vi "ConfigCalculateMinimalAcquisitionTime.vi"(7 "Single Pump Cycle Refresh Ratio":dbl, 9 "Loop Microscope Settings":string[][](array[string]), 10 "Positions":string[][](array[string]), 11 "Program":string[][](array[string])) -> (0 "Microscope Out":string[][](array[string]), 1 "Positions out":string[][](array[string]), 2 "Program out":string[][](array[string]), 3 "Time (Time Stamp)":timestamp)   [LabVIEW 2018, in "Config.lvlib"]
uses:
  Config.lvlib
  ContinuousLoop/ContinousLoop.lvlib
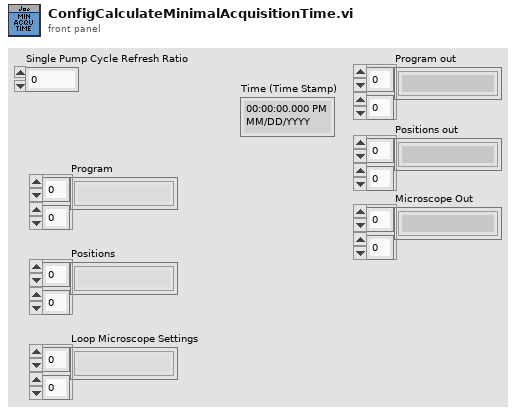
[diagram p1: front panel]
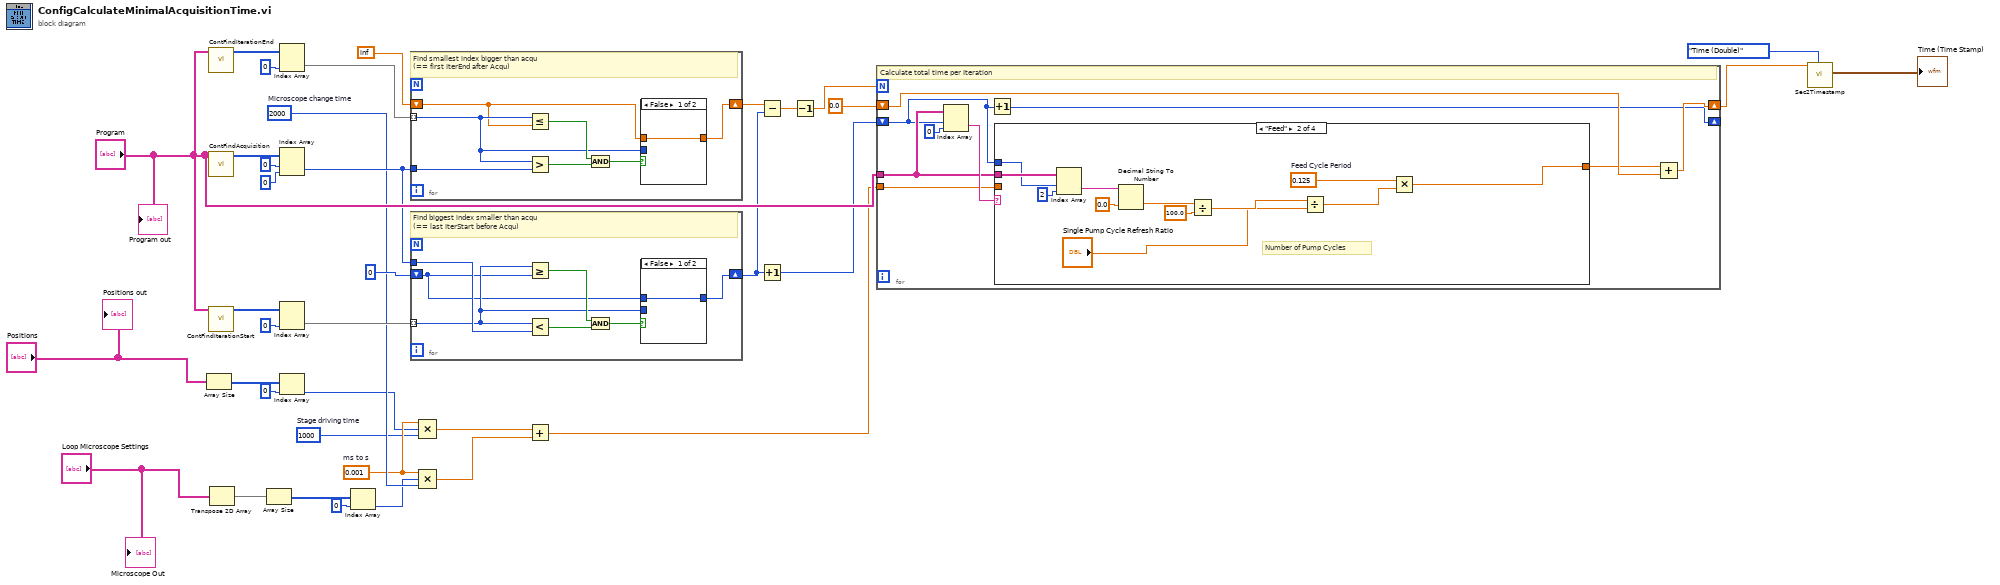
[diagram p0: block diagram]
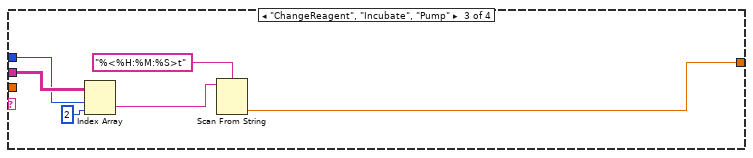
[diagram p3: hidden frame]
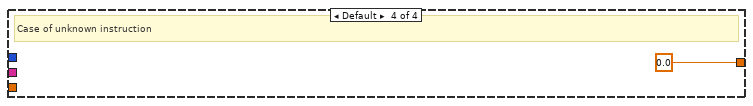
[diagram p4: hidden frame]
diagram:
  w11 = 0.001  # ms to s
  w15 = 2000  # Microscope change time
  w7 = 1000  # Stage driving time
  n1 = Array Size(array="Positions") -> (size(s)=w4:i32[])
  n2 = call "ContFindIterationEnd.vi"("Continuous Program in"="Program") -> ("Array out"=w19:i32[][])  [unwired: 10 in]
  n3 = call "ContFindAcquisition.vi"("ItemNames"="Program") -> ("Array"=w20:i32[][])  [unwired: 10 in]
  n4 = call "ContFindIterationStart.vi"("ItemNames"="Program") -> ("Array"=w17:i32[][])  [unwired: 10 in]
  n5 = Transpose 2D Array(2D array="Loop Microscope Settings") -> (transposed array=w2:string[][])
  n6 = Array Size(array=w2) -> (size(s)=w3:i32[])
  n7 = Index Array(array=w19, index (col)=0 ("index")) -> (element=w23:i32[])  [unwired: 1 in]
  n8 = Index Array(array=w20, index (row)=0 ("index"), index (col)=0 ("disabled index (col)")) -> (element=w25:i32)
  n9 = Index Array(array=w17, index (col)=0 ("index")) -> (element=w21:i32[])  [unwired: 1 in]
  n10 = Index Array(array=w4, index=0) -> (element=w1:i32)
  n11 = Index Array(array=w3, index=0) -> (element=w14:i32)
  n12 = for {
    tunnel: w23 -> [w39] mode=indexing
    tunnel: w25 -> [w44]
    shift-right: [w40] -> w26
    shift-left: inf -> [w38]
    # "Find smallest index bigger than acqu\n(== first IterEnd after Acqu)"
    n13 = Less Or Equal?(x=w39, y=w38) -> (x <= y?=w41:bool)
    n14 = Greater?(x=w39, y=w44) -> (0:w43:bool)
    n15 = And(x=w41, y=w43) -> (x .and. y?=w42:bool)
    n16 = case shown="False" w42 {
      tunnel: [w45 w46] -> w40
      tunnel: w39 -> [_ w46]
      tunnel: w38 -> [w45 _]
      frame False {
      }
      frame True {
      }
    }
  }
  n17 = for {
    tunnel: w21 -> [w48] mode=indexing
    tunnel: w25 -> [w53]
    shift-right: [w49] -> w29
    shift-left: 0 -> [w47]
    # "Find biggest index smaller than acqu\n(== last IterStart before Acqu)"
    n18 = Greater Or Equal?(x=w48, y=w47) -> (x >= y?=w50:bool)
    n19 = Less?(x=w48, y=w53) -> (x < y?=w52:bool)
    n20 = And(x=w50, y=w52) -> (x .and. y?=w51:bool)
    n21 = case shown="False" w51 {
      tunnel: [w54 w55] -> w49
      tunnel: w48 -> [_ w55]
      tunnel: w47 -> [w54 _]
      frame False {
      }
      frame True {
      }
    }
  }
  n22 = Compound Arithmetic op=MULTIPLY(w11, w1, w7) -> (w12:dbl)
  n23 = Compound Arithmetic op=MULTIPLY(w11, w14, w15) -> (w13:dbl)
  n24 = Add(x=w12, y=w13) -> (x+y=w33:dbl)
  n25 = Subtract(x=w26, y=w29) -> (x-y=w27:dbl)
  n26 = Increment(x=w29) -> (x+1=w30:i32)
  n27 = Decrement(x=w27) -> (x-1=w28:dbl)
  n28 = for {
    N: w28 -> [_]
    tunnel: "Program" -> [w61]
    shift-right: [w60] -> w32
    shift-left: 0.0 -> [w59]
    tunnel: w33 -> [w62]
    shift-right: [w56] -> _
    shift-left: w30 -> [w57]
    # "Calculate total time per Iteration"
    n29 = Index Array(array=w61, index (row)=w57, index (col)=0 ("disabled index (col)")) -> (element=w63:string)
    n30 = Increment(x=w57) -> (x+1=w56:i32)
    n31 = case shown="\"Feed\"" w63 {
      tunnel: w62 -> [w65 _ _ _]
      tunnel: [w65 w70 w78 0.0] -> w58
      tunnel: w61 -> [_ w72 w81 _]
      tunnel: w57 -> [_ w71 w79 _]
      frame "Acquire" {
      }
      frame "Feed" {
        w69 = 0.125  # Feed Cycle Period
        # "Number of Pump Cycles"
        n32 = Index Array(array=w72, index (row)=w71, index (col)=2 ("disabled index (col)")) -> (element=w76:string)
        n33 = Decimal String To Number(string=w76, default (0L)=0.0) -> (number=w74:dbl)  [unwired: 1 in, 1 out]
        n34 = Divide(x=w74, y=100.0) -> (x/y=w68:dbl)
        n35 = Divide(x=w68, y="Single Pump Cycle Refresh Ratio") -> (x/y=w73:dbl)
        n36 = Multiply(x=w69, y=w73) -> (x*y=w70:dbl)
      }
      frame "ChangeReagent", "Incubate", "Pump" {
        n37 = Index Array(array=w81, index (row)=w79, index (col)=2 ("disabled index (col)")) -> (element=w80:string)
        n38 = Scan From String(format string="%<%H:%M:%S>t", input string=w80) -> (output 1=w78:dbl)  [unwired: 3 in, 3 out]
      }
      frame Default {
        # "Case of unknown instruction"
      }
    }
    n39 = Add(x=w58, y=w59) -> (x+y=w60:dbl)
  }
  n40 = call "Sec2Timestamp.vi"("Input Selection"=enum32{"Time (Double)", "Time (Time Stamp)"}."Time (Double)", "Input Time (Double)"=w32) -> ("Time (Time Stamp)"=→"Time (Time Stamp)":timestamp)  [unwired: 7 in, 2 out]
  "Program out" <- "Program"
  "Positions out" <- "Positions"
  "Microscope Out" <- "Loop Microscope Settings"
